vi "GetDriverInfo.vi"(4 "error in (no error)":errorcluster) -> (0 "error out":errorcluster, 2 "libraryVersion":string, 3 "libraryName":string)   [LabVIEW 2018]
doc: "<B>GetDriverInfo</B> returns the name and version from the Windows DLL."
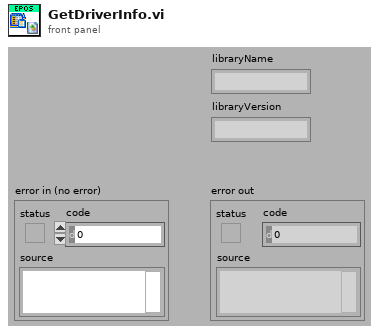
[diagram p1: front panel]
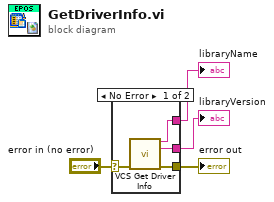
[diagram p0: block diagram]
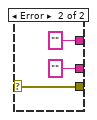
[diagram p2: hidden frame]
diagram:
  n1 = case shown="No Error" "error in (no error)" {
    selector: "error in (no error)" -> [w8 w11]
    tunnel: [w7 w11] -> w3
    tunnel: [w6 "" ("libraryName")] -> w2
    tunnel: [w5 "" ("libraryVersion")] -> w1
    frame No Error {
      n2 = call "VCS Get Driver Info.vi"("error in (no error)"=w8) -> ("libraryName"=w6:string, "libraryVersion"=w5:string, "error out"=w7:errorcluster)  [unwired: 12 in]
    }
    frame Error {
    }
  }
  "error out" <- w3
  "libraryName" <- w2
  "libraryVersion" <- w1
